vi "USB2XXXIICAM2321.vi"() -> ()   [LabVIEW 2010]
uses:
  PublicFiles/usb_device/USB2XXX.dll
panel:
  out "湿度/百分比":dbl
  out "温度/摄氏度":dbl
  out "湿度":dbl(slide) scale=0.0..100.0
  out "温度":dbl(slide) scale=0.0..100.0
  out "工作状态":bool
  in  "pConfig":T1
  in  "Channel Index":i32(ring) items=["CH0", "CH1", "CH2", "CH3", "CH4", "CH5", "CH6", "CH7"]
  in  "Device Index":i32(ring) items=["0", "1", "2", "3", "4", "5"]
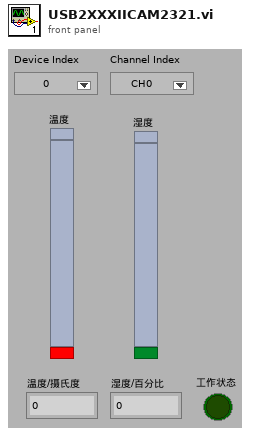
[diagram p1: front panel]
types:
  T1 = cluster{"ClockSpeedHz":u32, "OwnAddr":u16, "Master":u8, "AddrBits":u8, "EnablePu":u8}
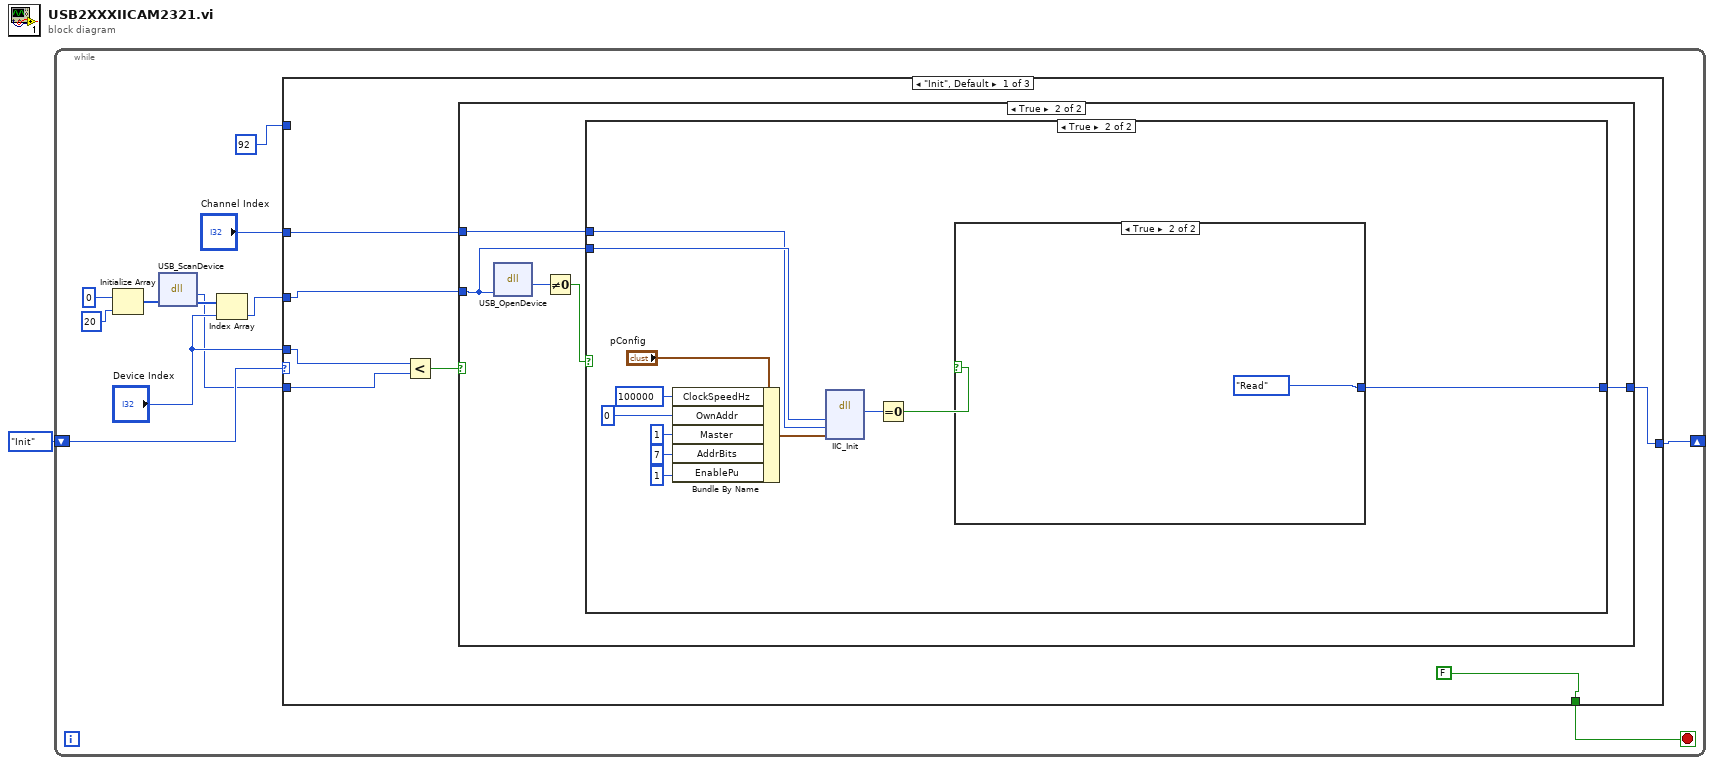
[diagram p0: block diagram]
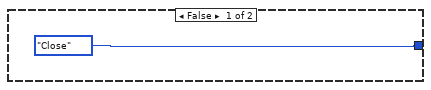
[diagram p2: hidden frame]
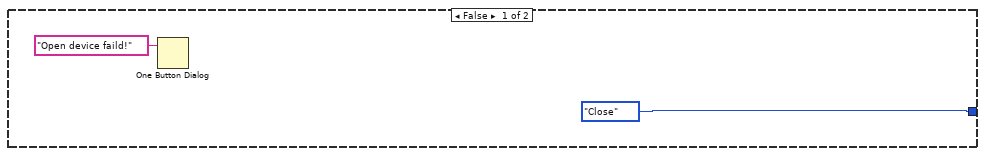
[diagram p3: hidden frame]
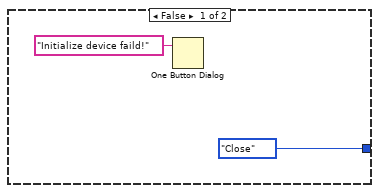
[diagram p4: hidden frame]
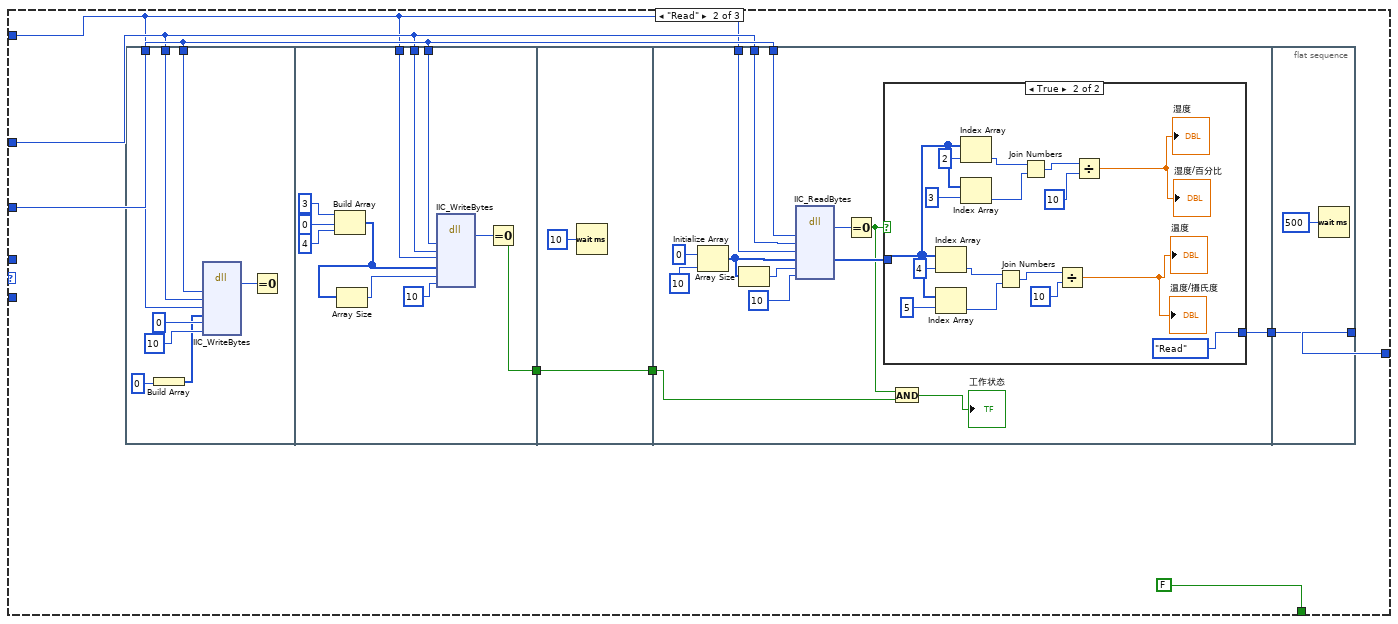
[diagram p5: hidden frame]
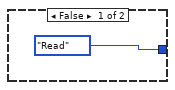
[diagram p6: hidden frame]
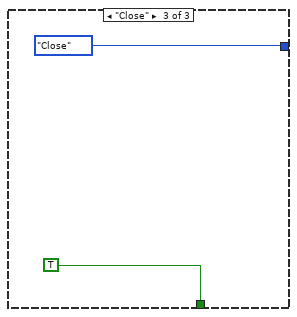
[diagram p7: hidden frame]
diagram:
  n1 = while {
    shift-right: [w12] -> _
    shift-left: enum16{"Init", "Read", "Close"}."Init" ("Enum") -> [w13]
    stop <- w9 stop-if-true
    n2 = Initialize Array(0, 20 ("dimension size")) -> (w8:i32[])
    n3 = dll-call lib="G:/OtherWork/USB2XXX_Example/trunk/Labview/PublicFiles/usb_device/USB2XXX.*" fn="USB_ScanDevice"("pDevNum"=w8) -> ("return type"=w2:i32, "pDevNum"=w5:i32[])  [unwired: 3 in, 2 out]
    n4 = Index Array(array=w5, index="Device Index") -> (element=w4:i32)
    n5 = case shown="\"Init\", Default" w13 {
      tunnel: [w19 w47 enum16{"Init", "Read", "Close"}."Close" ("Enum")] -> w12
      tunnel: w4 -> [w18 w50 _]
      tunnel: "Channel Index" -> [w17 w49 _]
      tunnel: i16 92 ("Slave Addr(Hex)") -> [_ w48 _]
      tunnel: [FALSE FALSE TRUE] -> w9
      tunnel: "Device Index" -> [w15 _ _]
      tunnel: w2 -> [w14 _ _]
      frame "Init", Default {
        n6 = Less?(x=w15, y=w14) -> (x < y?=w20:bool)
        n7 = case shown="True" w20 {
          tunnel: w18 -> [_ w23]
          tunnel: w17 -> [_ w24]
          tunnel: [enum16{"Init", "Read", "Close"}."Close" ("Enum") w22] -> w19
          frame False {
          }
          frame True {
            n8 = dll-call lib="G:/OtherWork/USB2XXX_Example/trunk/Labview/PublicFiles/usb_device/USB2XXX.*" fn="USB_OpenDevice"("DevIndex"=w23) -> (w26:u8)  [unwired: 4 in, 2 out]
            n9 = Not Equal To 0?(x=w26) -> (x != 0?=w25:bool)
            n10 = case shown="True" w25 {
              tunnel: w24 -> [_ w32]
              tunnel: w23 -> [_ w33]
              tunnel: [enum16{"Init", "Read", "Close"}."Close" ("Enum") w29] -> w22
              frame False {
                n11 = One Button Dialog(message="Open device faild!") -> ()  [unwired: 1 in, 1 out]
              }
              frame True {
                n12 = Bundle By Name(cluster="pConfig", "ClockSpeedHz"=u32 100000, "OwnAddr"=u16 0, "Master"=u8 1, "AddrBits"=u8 7, "EnablePu"=u8 1) -> (w39:T1)
                n13 = dll-call lib="G:/OtherWork/USB2XXX_Example/trunk/Labview/PublicFiles/usb_device/USB2XXX.*" fn="IIC_Init"("DevIndex"=w33, "IICIndex"=w32, "pConfig"=w39) -> (w31:i32)  [unwired: 6 in, 2 out]
                n14 = Equal To 0?(x=w31) -> (x = 0?=w30:bool)
                n15 = case shown="True" w30 {
                  tunnel: [enum16{"Init", "Read", "Close"}."Close" ("Enum") enum16{"Init", "Read", "Close"}."Read" ("Enum")] -> w29
                  frame False {
                    n16 = One Button Dialog(message="Initialize device faild!") -> ()  [unwired: 1 in, 1 out]
                  }
                  frame True {
                  }
                }
              }
            }
          }
        }
      }
      frame "Read" {
        n17 = flat-sequence {
          tunnel: w50 -> [w56]
          tunnel: w49 -> [w55]
          tunnel: w48 -> [w54]
          tunnel: w50 -> [w63]
          tunnel: w49 -> [w62]
          tunnel: w48 -> [w61]
          tunnel: [w60] -> w45
          tunnel: w45 -> [w71]
          tunnel: [w71] -> w44
          tunnel: w50 -> [w86]
          tunnel: w49 -> [w85]
          tunnel: w48 -> [w84]
          tunnel: [w76] -> w46
          tunnel: w44 -> [w73]
          tunnel: [w105] -> w47
          tunnel: w46 -> [w105]
          frame #0 {
            n18 = Build Array(u8 0 ("WriteLen")) -> (w53:u8[])
            n19 = dll-call lib="G:/OtherWork/USB2XXX_Example/trunk/Labview/PublicFiles/usb_device/USB2XXX.*" fn="IIC_WriteBytes"("DevIndex"=w56, "IICIndex"=w55, "SlaveAddr"=w54, "pWriteData"=w53, "WriteLen"=0, "TimeOutMs"=10) -> (w58:i32)  [unwired: 9 in, 2 out]
            n20 = Equal To 0?(x=w58) -> ()  [unwired: 1 out]
          }
          frame #1 {
            n21 = Build Array(u8 3, u8 0 ("element"), u8 4 ("element")) -> (w64:u8[])
            n22 = Array Size(array=w64) -> (size(s)=w70:i32)
            n23 = dll-call lib="G:/OtherWork/USB2XXX_Example/trunk/Labview/PublicFiles/usb_device/USB2XXX.*" fn="IIC_WriteBytes"("DevIndex"=w63, "IICIndex"=w62, "SlaveAddr"=w61, "pWriteData"=w64, "WriteLen"=w70, "TimeOutMs"=10) -> (w68:i32)  [unwired: 9 in, 2 out]
            n24 = Equal To 0?(x=w68) -> (x = 0?=w60:bool)
          }
          frame #2 {
            n25 = Wait (ms)(milliseconds to wait=u32 10) -> ()  [unwired: 1 out]
          }
          frame #3 {
            n26 = Initialize Array(u8 0 ("element"), 10 ("dimension size")) -> (w81:u8[])
            n27 = Array Size(array=w81) -> (size(s)=w80:i32)
            n28 = dll-call lib="G:/OtherWork/USB2XXX_Example/trunk/Labview/PublicFiles/usb_device/USB2XXX.*" fn="IIC_ReadBytes"("DevIndex"=w86, "IICIndex"=w85, "SlaveAddr"=w84, "pReadData"=w81, "ReadLen"=w80, "TimeOutMs"=10) -> (w78:i32, "pReadData"=w77:u8[])  [unwired: 8 in, 2 out]
            n29 = Equal To 0?(x=w78) -> (x = 0?=w74:bool)
            n30 = case shown="True" w74 {
              tunnel: w77 -> [_ w95]
              tunnel: [enum16{"Init", "Read", "Close"}."Read" ("Enum") enum16{"Init", "Read", "Close"}."Read" ("Enum")] -> w76
              frame False {
              }
              frame True {
                n31 = Index Array(array=w95, index=4) -> (element=w101:u8)
                n32 = Index Array(array=w95, index=5) -> (element=w100:u8)
                n33 = Index Array(array=w95, index=2) -> (element=w97:u8)
                n34 = Index Array(array=w95, index=3) -> (element=w96:u8)
                n35 = Join Numbers(hi=w101, lo=w100) -> ((hi.lo)=w92:u16)
                n36 = Join Numbers(hi=w97, lo=w96) -> ((hi.lo)=w94:u16)
                n37 = Divide(x=w92, y=u16 10) -> (x/y=→"温度/摄氏度" →"温度":dbl)
                n38 = Divide(x=w94, y=u16 10) -> (x/y=→"湿度/百分比" →"湿度":dbl)
              }
            }
            n39 = And(x=w74, y=w73) -> (x .and. y?=→"工作状态":bool)
          }
          frame #4 {
            n40 = Wait (ms)(milliseconds to wait=u32 500) -> ()  [unwired: 1 out]
          }
        }
      }
      frame "Close" {
      }
    }
  }
